vi "Add dllspec To Functions Prototypes.vi"(8 "Error In":errorcluster, 10 "dllspec token":string="EXAMPLE_DLL", 11 "input string":string="long lubo();\nint something else();\n\nvoid ugo(int a = 0);\n") -> (0 "Error Out":errorcluster, 3 "String":string)   [LabVIEW 2014]
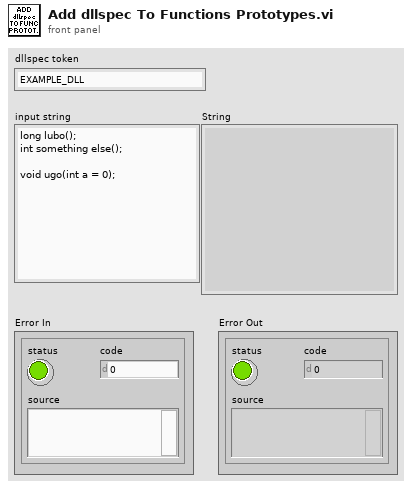
[diagram p1: front panel]
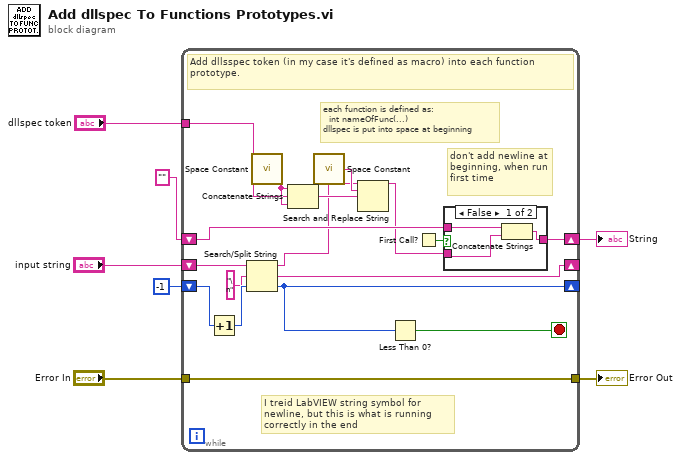
[diagram p0: block diagram]
diagram:
  n1 = while {
    tunnel: "Error In" -> [w16]
    shift-right: [w24] -> w3
    shift-left: "" -> [w23]
    shift-right: [w17] -> _
    shift-left: -1 ("offset of match") -> [w21]
    shift-right: [w20] -> _
    shift-left: "input string" -> [w22]
    tunnel: [w16] -> w4
    tunnel: "dllspec token" -> [w10]
    stop <- w18 stop-if-true
    # "don't add newline at beginning, when run first time"
    # "I treid LabVIEW string symbol for newline, but this is what is running correctly in the end"
    # "each function is defined as:\n  int nameOfFunc(...)\ndllspec is put into space at beginning"
    # "Add dllsspec token (in my case it's defined as macro) into each function prototype."
    n2 = Increment(x=w21) -> (x+1=w19:i32)
    n3 = Search/Split String(string=w22, search string/char (-)="\n", offset (0)=w19) -> (substring before match=w9:string, match + rest of string=w20:string, offset of match=w17:i32)
    n4 = call <vilib>:"Space Constant.vi"() -> ("String"=w13:string)
    n5 = Concatenate Strings(w13, w10, w13) -> (w12:string)
    n6 = call <vilib>:"Space Constant.vi"() -> ("String"=w11:string)
    n7 = Search and Replace String(input string=w9, search string=w11, replace string=w12) -> (result string=w8:string)  [unwired: 5 in, 3 out]
    n8 = Less Than 0?(x=w17) -> (x < 0?=w18:bool)
    n9 = First Call?() -> (First Call?: T/F=w14:bool)
    n10 = case shown="False" w14 {
      tunnel: [w27 w28] -> w24
      tunnel: w23 -> [w26 _]
      tunnel: w8 -> [w25 w28]
      frame False {
        n11 = Concatenate Strings(w26, w25) -> (w27:string)
      }
      frame True {
      }
    }
  }
  "Error Out" <- w4
  "String" <- w3
